vi "ReadSerial.vi"(8 "error in (no error)":errorcluster, 11 "VISA Refnum in":refnum<visa-resource-name>) -> (0 "error out":errorcluster, 2 "String":string, 3 "VISA Refnum out":refnum<visa-resource-name>)   [LabVIEW 2019]
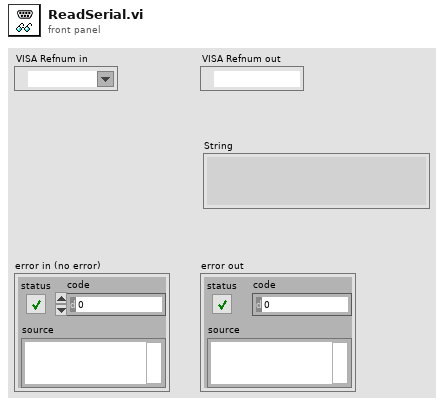
[diagram p1: front panel]
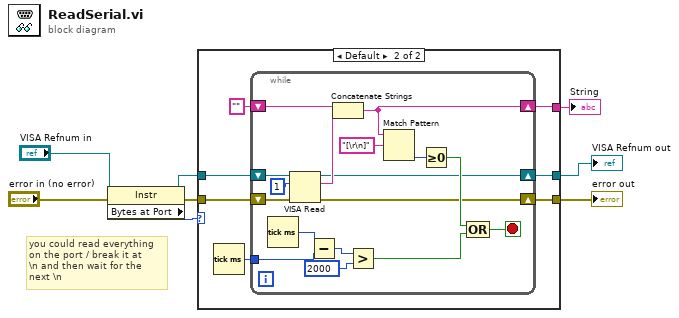
[diagram p0: block diagram]
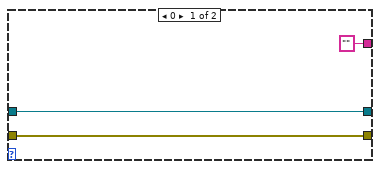
[diagram p2: hidden frame]
diagram:
  # "you could read everything\non the port / break it at\n\\n and then wait for the\nnext \\n"
  n1 = property class="Instr"(reference="VISA Refnum in", error in="error in (no error)") -> (reference out=w2:refnum<visa-resource-name>, error out=w4:errorcluster, "Bytes at Port"=w7:u32)
  n2 = case shown="Default" w7 {
    tunnel: w2 -> [w11 w18]
    tunnel: w4 -> [w10 w17]
    tunnel: [w10 w16] -> w5
    tunnel: [w11 w15] -> w6
    tunnel: ["" w12] -> w1
    frame 0 {
    }
    frame Default {
      n3 = Tick Count (ms)() -> (millisecond timer value=w13:u32)
      n4 = while {
        shift-right: [w19] -> w15
        shift-left: w18 -> [w35]
        shift-right: [w20] -> w16
        shift-left: w17 -> [w34]
        shift-right: [w30] -> w12
        shift-left: "" -> [w32]
        tunnel: w13 -> [w26]
        stop <- w21 stop-if-true
        n5 = Tick Count (ms)() -> (millisecond timer value=w27:u32)
        n6 = VISA Read(VISA resource name=w35, byte count=u32 1, error in (no error)=w34) -> (VISA resource name out=w19:refnum<visa-resource-name>, read buffer=w31:string, error out=w20:errorcluster)  [unwired: 1 out]
        n7 = Subtract(x=w27, y=w26) -> (x-y=w25:u32)
        n8 = Concatenate Strings(w32, w31) -> (w30:string)
        n9 = Greater?(x=w25, y=u32 2000 ("byte count")) -> (0:w23:bool)
        n10 = Match Pattern(string=w30, regular expression="[\r\n]") -> (offset past match=w28:i32)  [unwired: 1 in, 3 out]
        n11 = Greater Or Equal To 0?(x=w28) -> (x >= 0?=w22:bool)
        n12 = Compound Arithmetic op=OR(w22, w23) -> (w21:bool)
      }
    }
  }
  "VISA Refnum out" <- w6
  "error out" <- w5
  "String" <- w1
